vi "Emballage_BDD_recherche_correspondance.vi"(8 "Error in":errorcluster caption="Error in (no error)", 10 "Chaîne":string, 11 "Tableau_IN":string[][](array[string])) -> (0 "Error out":errorcluster, 2 "résultat":bool, 3 "élément":i32)   [LabVIEW 2020]
uses:
  Modules/FS/60_FS_Controles/60_FS_SetGet.ctl
panel:
  out "Tableau_designation":i32[](array[numeric])
  out "Tableau_suffixe":i32[](array[numeric])
  out "Tableau_No_Valve_FAS":i32[](array[numeric])
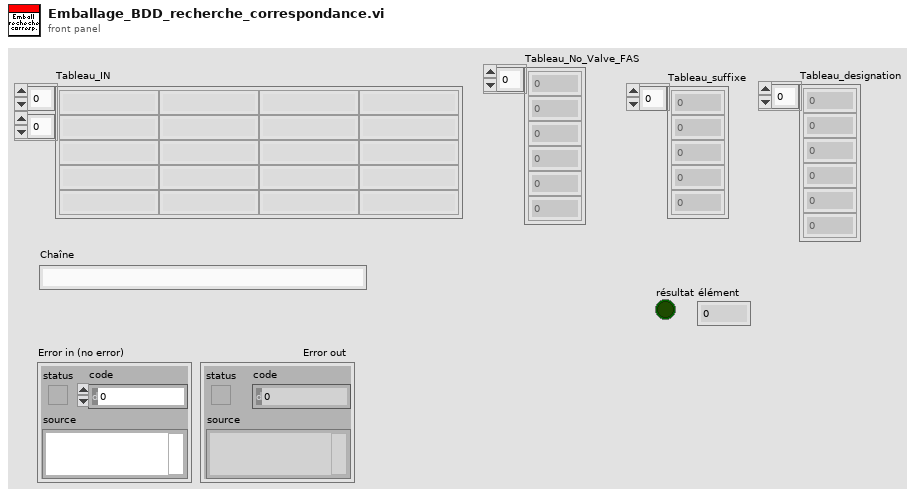
[diagram p1: front panel]
types:
  T1 = typedef "60_FS_SetGet.ctl" = enum16{"set", "get"}
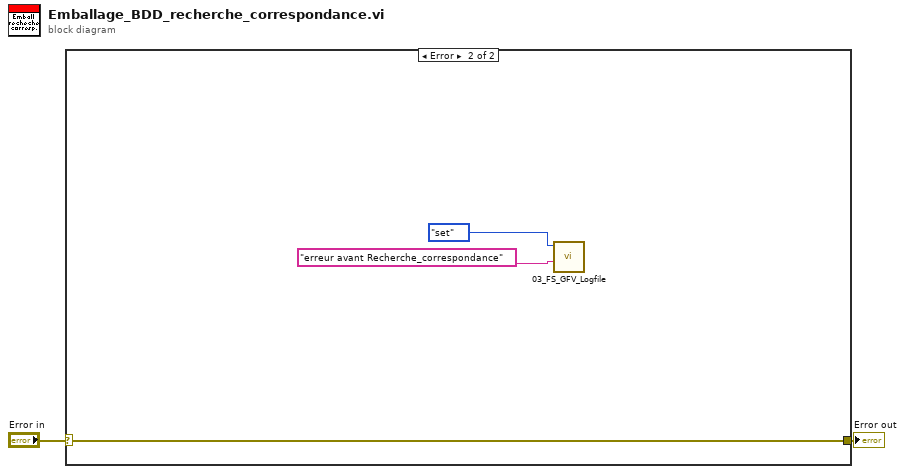
[diagram p0: block diagram]
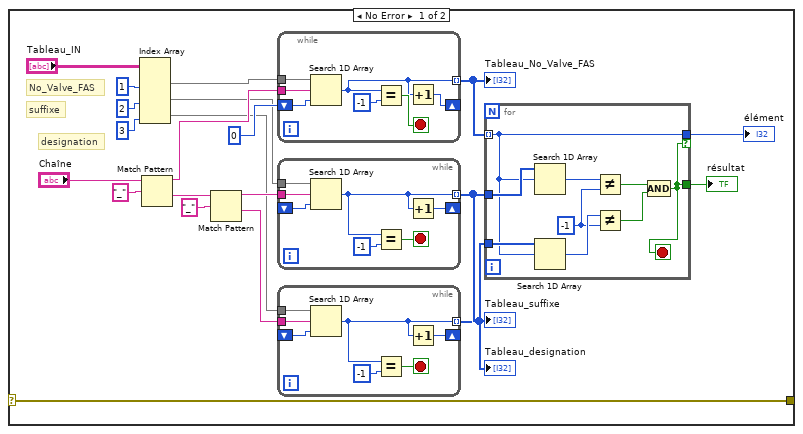
[diagram p2: hidden frame]
diagram:
  n1 = case shown="Error" "Error in" {
    selector: "Error in" -> [w3 w56]
    tunnel: [w3 w56] -> w1
    frame No Error {
      # "designation"
      # "suffixe"
      # "No_Valve_FAS"
      n2 = Index Array(array="Tableau_IN", index (col) #1=1 ("indice désactivé (col)"), index (col) #2=2 ("indice (col)"), index (col) #3=3 ("indice (col)")) -> (element #1=w17:string[], element #2=w12:string[], element #3=w10:string[])  [unwired: 3 in]
      n3 = Match Pattern(string="Chaîne", regular expression="_" ("expression régulière")) -> (before substring=w16:string, after substring=w14:string)  [unwired: 1 in, 2 out]
      n4 = Match Pattern(string=w14, regular expression="_" ("expression régulière")) -> (before substring=w11:string, after substring=w9:string)  [unwired: 1 in, 2 out]
      n5 = while {
        tunnel: w17 -> [w53]
        tunnel: w16 -> [w52]
        shift-right: [w47] -> _
        shift-left: 0 -> [w51]
        tunnel: [w48] -> w8 mode=indexing
        stop <- w50 stop-if-true
        n6 = Search 1D Array(1D array=w53, element=w52, start index (0)=w51) -> (index of element=w48:i32)
        n7 = Equal?(x=w48, y=-1) -> (x = y?=w50:bool)
        n8 = Increment(x=w48) -> (x+1=w47:i32)
      }
      "Tableau_No_Valve_FAS" <- w8
      n9 = while {
        tunnel: w12 -> [w46]
        tunnel: w11 -> [w45]
        shift-right: [w40] -> _
        shift-left: _ -> [w44]
        tunnel: [w41] -> w7 mode=indexing
        stop <- w43 stop-if-true
        n10 = Search 1D Array(1D array=w46, element=w45, start index (0)=w44) -> (index of element=w41:i32)
        n11 = Equal?(x=w41, y=-1) -> (x = y?=w43:bool)
        n12 = Increment(x=w41) -> (x+1=w40:i32)
      }
      "Tableau_suffixe" <- w7
      n13 = while {
        tunnel: w10 -> [w39]
        tunnel: w9 -> [w38]
        shift-right: [w33] -> _
        shift-left: _ -> [w37]
        tunnel: [w34] -> w6 mode=indexing
        stop <- w36 stop-if-true
        n14 = Search 1D Array(1D array=w39, element=w38, start index (0)=w37) -> (index of element=w34:i32)
        n15 = Equal?(x=w34, y=-1) -> (x = y?=w36:bool)
        n16 = Increment(x=w34) -> (x+1=w33:i32)
      }
      "Tableau_designation" <- w6
      n17 = for {
        tunnel: w8 -> [w25] mode=indexing
        tunnel: w7 -> [w32]
        tunnel: w6 -> [w31]
        tunnel: [w24] -> w5
        tunnel: [w25] -> w4 if=w24
        stop <- w24 stop-if-true
        w26 = -1 ("y")
        n18 = Search 1D Array(1D array=w32, element=w25) -> (index of element=w30:i32)  [unwired: 1 in]
        n19 = Search 1D Array(1D array=w31, element=w25) -> (index of element=w29:i32)  [unwired: 1 in]
        n20 = Not Equal?(x=w30, y=w26) -> (x != y?=w28:bool)
        n21 = Not Equal?(x=w29, y=w26) -> (x != y?=w27:bool)
        n22 = Compound Arithmetic op=AND ("Opérateur arithmétique")(w28, w27) -> (w24:bool)
      }
      "résultat" <- w5
      "élément" <- w4
    }
    frame Error {
      n23 = call "03_FS_GFV_Logfile.vi"("Chaîne"="erreur avant Recherche_correspondance", "States"=60_FS_SetGet."set") -> ()  [unwired: 8 in, 2 out]
    }
  }
  "Error out" <- w1
